vi "Read id.vi"(8 "error in (no error)":errorcluster, 11 "data_node in":refnum<class "data_node.lvclass">) -> (0 "error out":errorcluster, 2 "id":string, 3 "data_node out":refnum<class "data_node.lvclass">)   [LabVIEW 2020, in "data_node.lvclass"]
uses:
  data_node.lvclass
  data_node.lvclass/data_node.ctl
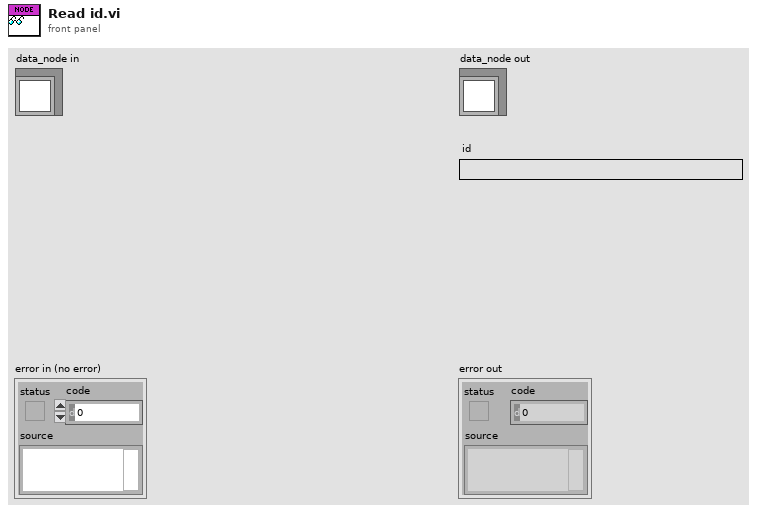
[diagram p1: front panel]
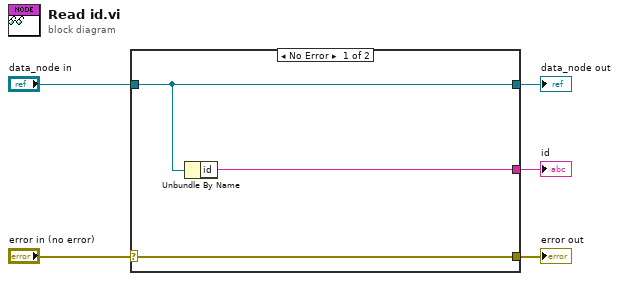
[diagram p0: block diagram]
diagram:
  n1 = case shown="No Error" "error in (no error)" {
    selector: "error in (no error)" -> [w8 w9]
    tunnel: [w8 w9] -> w4
    tunnel: [w7 w10] -> w2
    tunnel: "data_node in" -> [w7 w10]
    tunnel: [w6 _] -> w1
    frame No Error {
      n2 = Unbundle By Name(w7) -> ("id"=w6:string)
    }
    frame Error {
    }
  }
  "error out" <- w4
  "data_node out" <- w2
  "id" <- w1
